vi "PilotPlant.vi"() -> ()   [LabVIEW 2015]
uses:
  <vilib>/addons/control/pid/NI_PID_pid.lvlib
  <vilib>/addons/control/pid/pid.llb/PID (DBL).vi
  state.ctl
  calcDoseorGetGraph.ctl
  data ave state.ctl
  Sensor buffer command.ctl
  file paths.ctl
  ini.ctl
  data channels.ctl
  coagbuffer.ctl
  model type.ctl
  Manual or Auto.ctl
  setpoints.ctl
  backwash.ctl
  coag.ctl
panel:
  in  "Tab Control":enum32{"Graphs", "Controls", "About"}(tab)
  out "coag":cluster{"time":timestamp[], "all coag in":dbl[]}(graph)
  out "Misc":cluster{timestamp[], dbl[]}[](graph)
  out "Turbidities":cluster{timestamp[], dbl[]}[](graph)
  out "Sludge valve":dbl(graph)
  out "Plant flow valve":dbl(graph)
  in  "data channel":T1
  out "recent data":dbl[](array[numeric])
  in  "setpoints":T2={"graph data interval (s)"=100.0, "sludge flow [L/s]"=0.0, "plant flow [L/s]"=0.05, "Plant Flow PID "={"proportional gain (Kc)"=0.05, "integral time (Ti, min)"=1.0, "derivative time (Td, min)"=0.01}, "Sludge PID "={"proportional gain (Kc)"=0.07, "integral time (Ti, min)"=1.0, "derivative time (Td, min)"=0.01}, "backwash"={"Filtered quality target [NTU]"=0.3, "min filtration time [s]"=600.0, "Ripen time [s]"=600.0}, "Coagulant"={"flocculator volume (L)"=0.0, "clarifier volume (L)"=0.0, "dose updates per HRT"=100, "target clarified turbidity (NTU)"=0.3, "Coagulant mode"=enum."manual", "Coag dose [mg/L]"=0.0, "pump mL/rev"=0.0, "clarifier flow [L/s]"=0.5, "min Coag dose [mg/L]"=0.0, "max Coag dose [mg/L]"=0.0, "Steps"=3, "HRT response delay"=1, "Ku*"=1.0}} {"Coagulant"."HRT response delay" min=1 max=10 step=1; "Coagulant"."Steps" min=3 step=1; "Coagulant"."clarifier flow [L/s]" min=0.0001 max=1.0 step=0.0001; "Coagulant"."target clarified turbidity (NTU)" min=0.1 max=5.0 step=0.01; "Coagulant"."dose updates per HRT" min=1 max=100 step=1; "Sludge PID"."derivative time (Td, min)" format="%.3f"; "Sludge PID"."integral time (Ti, min)" format="%.3f"; "Sludge PID"."proportional gain (Kc)" format="%.3f"; "Plant Flow PID"."derivative time (Td, min)" format="%.3f"; "Plant Flow PID"."integral time (Ti, min)" format="%.3f"; "Plant Flow PID"."proportional gain (Kc)" format="%.3f"; "plant flow [L/s]" min=0.05 max=1.0 step=0.05; "sludge flow [L/s]" min=0.0 max=0.05 step=0.001; "graph data interval (s)" min=1 max=1000 step=1}
  in  "Sludge valve [V]":dbl(slide)=1.5 scale=0.0..5.0
  in  "Sludge control":bool
  out "coag pump In Range?":bool
  out "coag model":T5
  in  "backwash [ON/OFF]":bool
  out "Last backwash":timestamp
  in  "Backwash control":T6
  out "error out":errorcluster
  out "total HRT":dbl
  out "coag dose [mg/L]":dbl
  out "rpm":dbl
  in  "channel":T1=enum."raw [NTU]"
  out "stopping":bool
  out "data labels":string[](array[string])
  in  "Shut Down":bool
  # "min"
  # "max"
  # "The coaglog saves the coagulant and turbidity values for that particular time. There is no offset to correct for HRT."
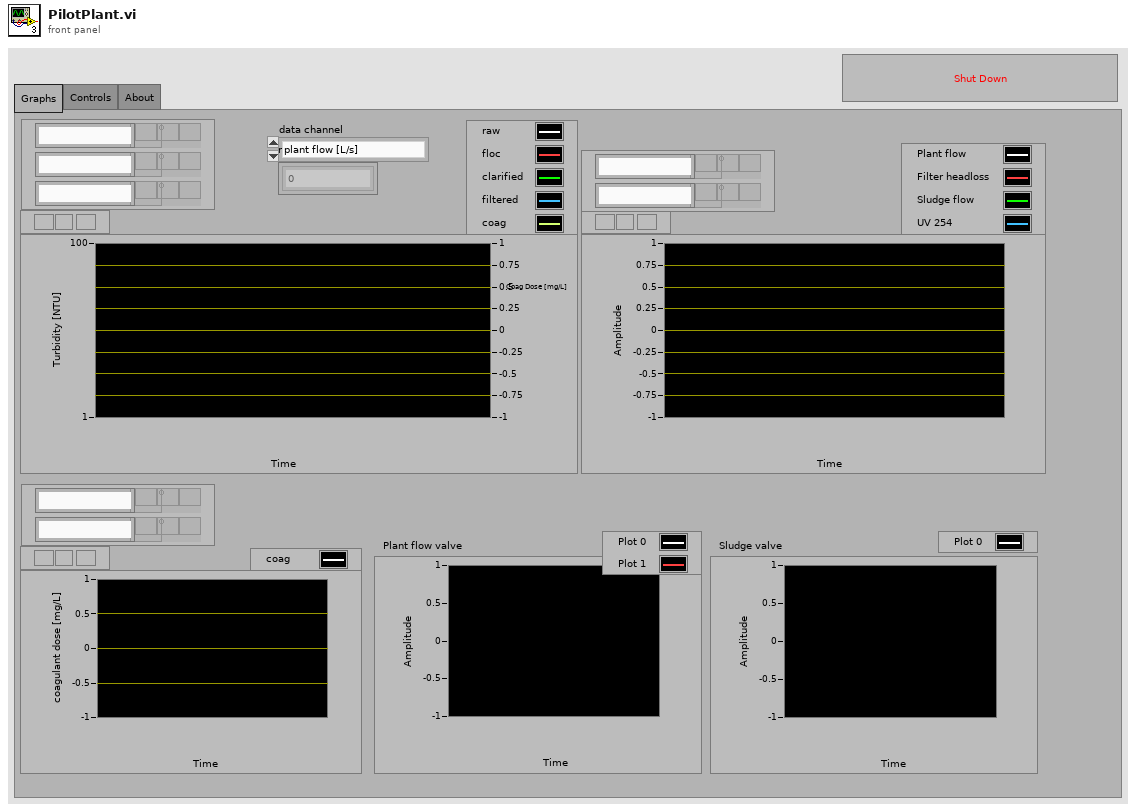
[diagram p1: front panel]
types:
  T1 = typedef "data channels.ctl" = enum16{"plant flow [L/s]", "Head Loss [m]", "sludge flow [L/s]", "UV 254", "raw [NTU]", "floc sed [NTU]", "clarified [NTU]", "filtered [NTU]"}
  T2 = typedef "setpoints.ctl" = cluster{"graph data interval (s)":sgl, "sludge flow [L/s]":dbl, "plant flow [L/s]":dbl, "Plant Flow PID ":cluster{"proportional gain (Kc)":dbl, "integral time (Ti, min)":dbl, "derivative time (Td, min)":dbl}, "Sludge PID ":cluster{"proportional gain (Kc)":dbl, "integral time (Ti, min)":dbl, "derivative time (Td, min)":dbl}, "backwash":T3, "Coagulant":T4}
  T3 = typedef "backwash.ctl" = cluster{"Filtered quality target [NTU]":dbl, "min filtration time [s]":dbl, "Ripen time [s]":dbl}
  T4 = typedef "coag.ctl" = cluster{"flocculator volume (L)":dbl, "clarifier volume (L)":dbl, "dose updates per HRT":u16, "target clarified turbidity (NTU)":dbl, "Coagulant mode":T5, "Coag dose [mg/L]":dbl, "pump mL/rev":dbl, "clarifier flow [L/s]":dbl, "min Coag dose [mg/L]":dbl, "max Coag dose [mg/L]":dbl, "Steps":u16, "HRT response delay":u32, "Ku*":dbl}
  T5 = typedef "model type.ctl" = enum16{"manual", "ramp", "simple corrector", "linear regression"}
  T6 = typedef "Manual or Auto.ctl" = enum16{"Manual", "Automatic"}
  T7 = typedef "file paths.ctl" = enum16{"read paths", "close"}
  T8 = typedef "ini.ctl" = enum16{"write", "read"}
  T9 = typedef "data ave state.ctl" = enum16{"Initialize", "Process data"}
  T10 = typedef "state.ctl" = enum16{"Initialize", "Process data", "Close"}
  T11 = typedef "Sensor buffer command.ctl" = enum16{"set buffer size", "write", "refill buffer", "read recent", "read all", "clear"}
  T12 = typedef "calcDoseorGetGraph.ctl" = enum16{"calculate dose", "read graph"}
  T13 = typedef "coagbuffer.ctl" = enum16{"set buffer size", "write", "refill buffer", "read recent", "read all", "clear", "overwrite"}
  T14 = typedef "data cluster.ctl" = cluster{"floc sed turbidity (NTU)":dbl, "Raw turbidity (NTU)":dbl, "flow rate (L/s)":dbl, "time":timestamp}
  T15 = cluster{"proportional gain (Kc)":dbl, "integral time (Ti, min)":dbl, "derivative time (Td, min)":dbl}
  T16 = cluster{"time":timestamp[], "all coag in":dbl[]}[]
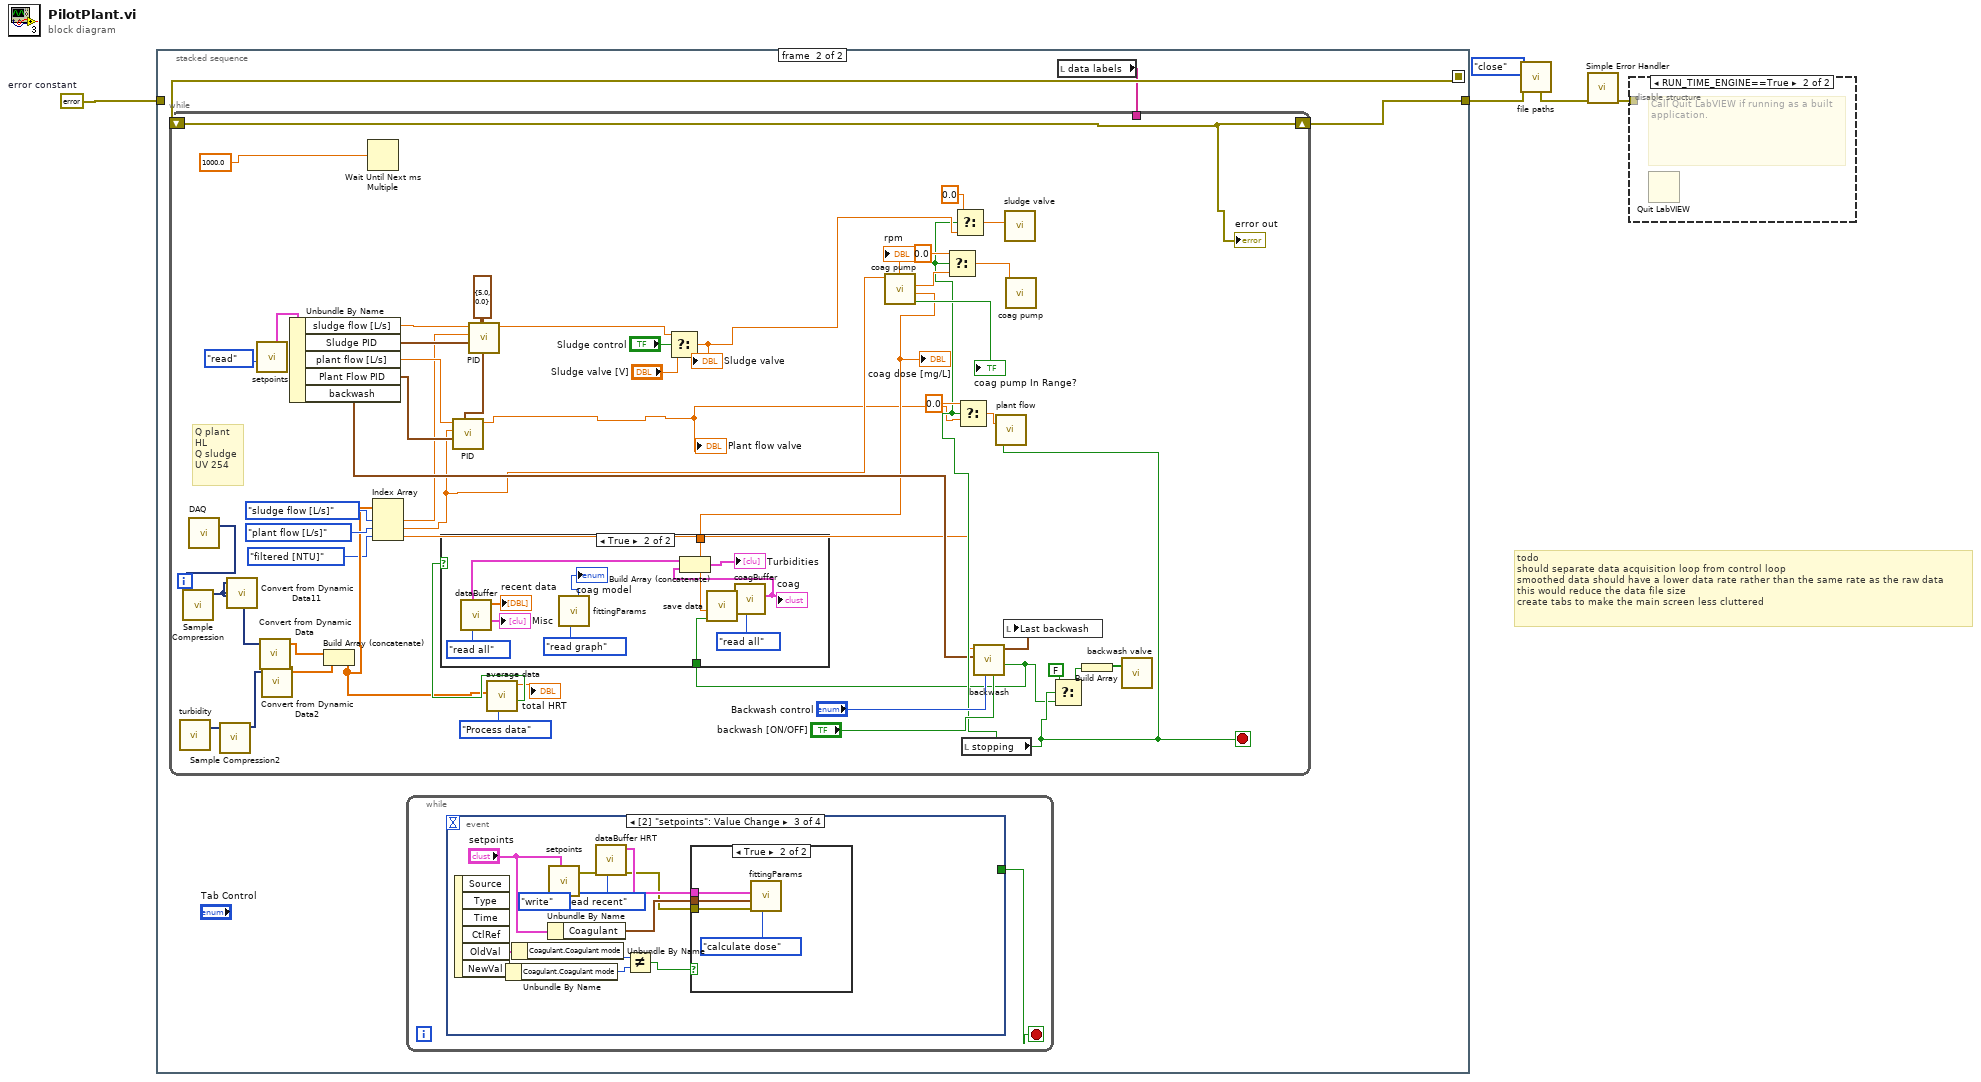
[diagram p0: block diagram]
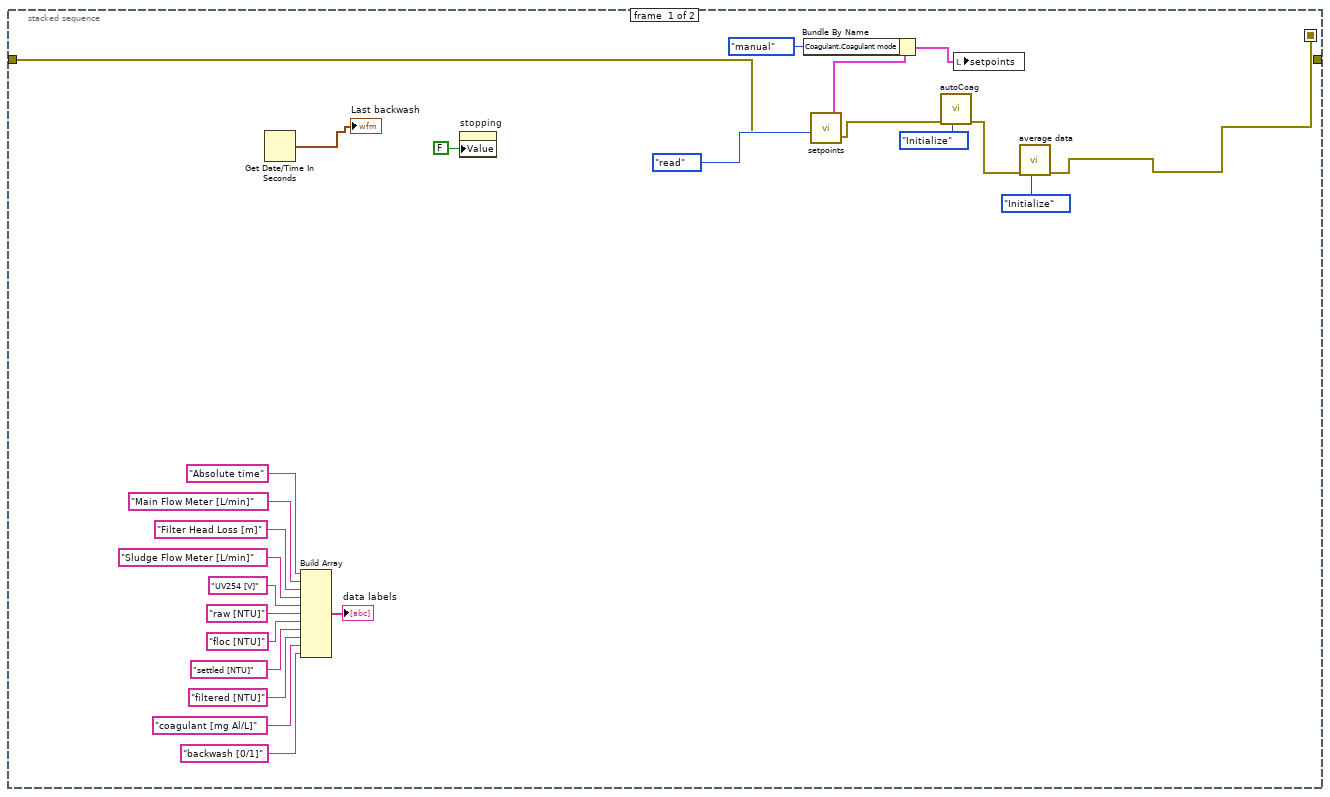
[diagram p2: hidden frame]
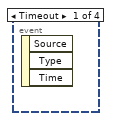
[diagram p3: hidden frame]
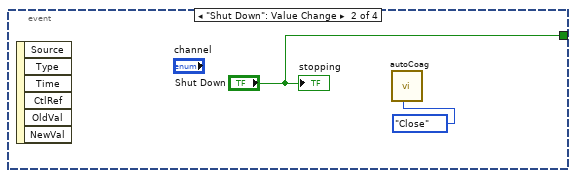
[diagram p4: hidden frame]
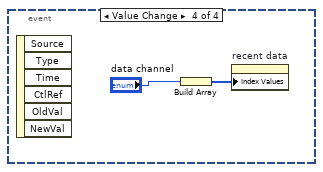
[diagram p6: hidden frame]
diagram:
  w5 = errorcluster {"status"=FALSE, "code"=0, "source"=""}  # error constant
  # "todo\nshould separate data acquisition loop from control loop\nsmoothed data should have a lower data rate rather than the same rate as the raw data\nthis would reduce the data file size\ncreate tabs to make the main screen less cluttered"
  n1 = stacked-sequence {
    seq-local: [w9 _] -> [_ w32]
    tunnel: w5 -> [w12 _]
    tunnel: [_ w30] -> w2
    frame #0 {
      n2 = Get Date/Time In Seconds() -> (seconds since 1Jan1904=→"Last backwash":timestamp)
      n3 = Build Array("Absolute time", "Main Flow Meter [L/min]", "Filter Head Loss [m]", "Sludge Flow Meter [L/min]", "UV254 [V]" ("element"), "raw [NTU]", "floc [NTU]", "settled [NTU]", "filtered [NTU]" ("element"), "coagulant [mg Al/L]" ("element"), "backwash [0/1]" ("element")) -> (→"data labels":string[])
      n4 = property on="stopping" class="Bool (strict)"("Value"=FALSE ("stopping")) -> ()  [unwired: 2 in, 2 out]
      n5 = call "setpoints.vi"("error in (no error)"=w12, "ini"=ini."read") -> ("error out"=w11:errorcluster, "Setpoints out"=w8:T2)  [unwired: 8 in]
      n6 = Bundle By Name(cluster=w8, "Coagulant.Coagulant mode"=model_type."manual") -> (w7:T2)
      n7 = call "autoCoag.vi"("state"=state."Initialize" ("Enum"), "error in (no error)"=w11) -> ("error out"=w14:errorcluster)  [unwired: 7 in, 2 out]
      n8 = local write "setpoints"(w7) -> ()
      n9 = call "average data.vi"("state"=data_ave_state."Initialize", "error in (no error)"=w14) -> ("error out"=w9:errorcluster)  [unwired: 5 in, 4 out]
    }
    frame #1 {
      n10 = while {
        stop <- w33 stop-if-true
        n11 = event shown="[2] \"setpoints\": Value Change" {
          selector: _ -> [_ _ _ _]
          dyn-events: _ -> [_ _ _ _]
          timeout: _ -> [_ _ _ _]
          tunnel: [_ "Shut Down" _ _] -> w33
          event Timeout {
            n12 = event-data() -> ()  [unwired: 1 in, 3 out]
          }
          event "Shut Down": Value Change {
            n13 = event-data() -> ()  [unwired: 1 in, 6 out]
            n14 = call "autoCoag.vi"("state"=state."Close" ("Enum")) -> ()  [unwired: 8 in, 3 out]
            "stopping" <- "Shut Down"
          }
          event Value Change {
            n15 = event-data() -> ("OldVal"=w39:T2, "NewVal"=w40:T2)  [unwired: 1 in, 4 out]
            n16 = Unbundle By Name(w40) -> ("Coagulant.Coagulant mode"=w37:T5)
            n17 = Unbundle By Name(w39) -> ("Coagulant.Coagulant mode"=w38:T5)
            n18 = Unbundle By Name("setpoints") -> ("Coagulant"=w45:T4)
            n19 = call "setpoints.vi"("setpoints"="setpoints", "ini"=ini."write") -> ("error out"=w42:errorcluster)  [unwired: 8 in, 1 out]
            n20 = call "dataBuffer HRT.vi"("command"=Sensor_buffer_command."read recent", "error in (no error)"=w42) -> ("error out"=w41:errorcluster, "recent data"=w44:T14)  [unwired: 6 in, 2 out]
            n21 = Not Equal?(x=w38, y=w37) -> (x != y?=w36:bool)
            n22 = case shown="True" w36 {
              tunnel: w45 -> [_ w51]
              tunnel: w44 -> [_ w49]
              tunnel: w41 -> [_ w48]
              frame False {
              }
              frame True {
                n23 = call "fittingParams.vi"("read/write"=calcDoseorGetGraph."calculate dose", "error in (no error)"=w48, "Coagulant"=w51, "averaged data"=w49) -> ()  [unwired: 5 in, 3 out]
              }
            }
          }
          event Value Change {
            n24 = event-data() -> ()  [unwired: 1 in, 6 out]
            n25 = Build Array("data channel") -> (w52:T1[])
            n26 = property on="recent data" class="Arr (strict)"("Index Values"=w52) -> ()  [unwired: 2 in, 2 out]
          }
        }
      }
      n27 = local read "data labels"() -> (w31:string[])
      n28 = while {
        shift-right: [w67] -> w30
        shift-left: w32 -> [w67]
        tunnel: w31 -> [_]
        stop <- w84 stop-if-true
        w97 = cluster{"output high":dbl, "output low":dbl} {"output high"=5.0, "output low"=0.0} ("output range")
        # "Q plant\nHL\nQ sludge\nUV 254"
        n29 = call "turbidity"() -> ("data"=w70:dynamicdata)  [unwired: 17 in, 2 out]
        n30 = call "DAQ"() -> ("data"=w71:dynamicdata)  [unwired: 17 in, 2 out]
        n31 = call "Sample Compression"("Signals"=w71) -> ("Mean"=w66:dynamicdata)  [unwired: 8 in, 2 out]
        n32 = call "Sample Compression2"("Signals"=w70) -> ("Mean"=w61:dynamicdata)  [unwired: 8 in, 2 out]
        n33 = call "Convert from Dynamic Data11"("Dynamic Data Type"=w66) -> ()  [unwired: 3 in, 1 out]
        n34 = call "setpoints.vi"("ini"=ini."read") -> ("Setpoints out"=w68:T2)  [unwired: 9 in, 1 out]
        n35 = call "Convert from Dynamic Data"("Dynamic Data Type"=w66) -> ("Array"=w82:dbl[])  [unwired: 3 in]
        n36 = call "Convert from Dynamic Data2"("Dynamic Data Type"=w61) -> ("Array"=w81:dbl[])  [unwired: 3 in]
        n37 = Unbundle By Name(w68) -> ("sludge flow [L/s]"=w77:dbl, "Sludge PID"=w76:T15, "plant flow [L/s]"=w75:dbl, "Plant Flow PID"=w74:T15, "backwash"=w73:T3)
        n38 = Build Array (concatenate)(w82, w81) -> (w60:dbl[])
        n39 = Wait Until Next ms Multiple(millisecond multiple=1000.0 ("y")) -> ()  [unwired: 1 out]
        n40 = Index Array(array=w60, index #1=data_channels."sludge flow [L/s]" ("channel"), index #2=data_channels."plant flow [L/s]" ("channel"), index #3=data_channels."filtered [NTU]" ("channel")) -> (element #1=w63:dbl, element #2=w62:dbl, element #3=w58:dbl)
        n41 = call-poly <vilib>:"PID.vi"("output range"=w97, "PID gains"=w74, "process variable"=w62, "setpoint"=w75) -> ("output"=w55:dbl)  [unwired: 6 in, 1 out]
        "Plant flow valve" <- w55
        n42 = call-poly <vilib>:"PID.vi"("output range"=w97, "PID gains"=w76, "process variable"=w63, "setpoint"=w77) -> ("output"=w98:dbl)  [unwired: 6 in, 1 out]
        n43 = call "average data.vi"("state"=data_ave_state."Process data", "data input"=w60) -> ("new interval"=w78:bool, "total HRT"=→"total HRT":dbl)  [unwired: 5 in, 3 out]
        n44 = Select(t=w98, s="Sludge control", f="Sludge valve [V]") -> (s? t:f=w88:dbl)
        "Sludge valve" <- w88
        n45 = call "coag pump.vi"("plant flow [L/s]"=w62) -> ("In Range?"=→"coag pump In Range?":bool, "coag dose [mg/L]"=w57:dbl, "pump [V]"=w93:dbl, "rpm"=→"rpm":dbl)  [unwired: 6 in, 1 out]
        "coag dose [mg/L]" <- w57
        n46 = local read "stopping"() -> (w84:bool)
        n47 = Select(t=0.0, s=w84, f=w93) -> (s? t:f=w92:dbl)
        n48 = Select(t=0.0, s=w84, f=w88) -> (s? t:f=w87:dbl)
        n49 = Select(t=0.0, s=w84, f=w55) -> (s? t:f=w91:dbl)
        n50 = call "backwash.vi"("Manual override"="backwash [ON/OFF]", "Backwash control"="Backwash control", "backwash"=w73, "Filtered Turbidity"=w58) -> ("backwashing?"=w56:bool, "last backwash"=w99:timestamp)  [unwired: 5 in, 1 out]
        n51 = case shown="True" w78 {
          tunnel: w57 -> [_ w109]
          tunnel: w56 -> [_ w108]
          frame False {
          }
          frame True {
            n52 = call "dataBuffer.vi"("command"=Sensor_buffer_command."read all") -> ("recent data"=→"recent data":dbl[], "misc graph"=→"Misc":cluster{timestamp[], dbl[]}[], "turbidity"=w112:cluster{timestamp[], dbl[]}[])  [unwired: 5 in, 3 out]
            n53 = call "fittingParams.vi"("read/write"=calcDoseorGetGraph."read graph") -> ("coag model"=→"coag model":T5)  [unwired: 8 in, 2 out]
            n54 = call "save data.vi"("backwashing?"=w108, "coagulant dose"=w109) -> ()  [unwired: 10 in]
            n55 = call "coagBuffer.vi"("command"=coagbuffer."read all") -> ("all data out"=w103:cluster{"time":timestamp[], "all coag in":dbl[]})  [unwired: 8 in, 2 out]
            "coag" <- w103
            n56 = Build Array (concatenate)(w112, w103) -> (→"Turbidities":T16)
          }
        }
        n57 = call "plant flow"("data"=w91, "stop (T)"=w84) -> ()  [unwired: 16 in, 2 out]
        n58 = local write "Last backwash"(w99) -> ()
        n59 = call "sludge valve"("data"=w87) -> ()  [unwired: 17 in, 2 out]
        n60 = call "coag pump"("data"=w92) -> ()  [unwired: 17 in, 2 out]
        n61 = Select(t=FALSE, s=w84, f=w56) -> (s? t:f=w85:bool)
        n62 = Build Array(w85) -> (w102:bool[])
        n63 = call "backwash valve"("data"=w102) -> ()  [unwired: 17 in, 2 out]
        "error out" <- w67
      }
    }
  }
  n64 = call "file paths.vi"("error in (no error)"=w2, "file path control"=file_paths."close") -> ("error out"=w1:errorcluster)  [unwired: 6 in, 3 out]
  n65 = call <vilib>:"Simple Error Handler.vi"("error in (no error)"=w1) -> ("error out"=w4:errorcluster)  [unwired: 4 in, 4 out]
  n66 = disable-structure shown="RUN_TIME_ENGINE==True" {
    disable-tunnel: w4 -> [_ _]
    frame condition #0 (active) {
    }
    frame condition #1 {
      # "Call Quit LabVIEW if running as a built application."
      n67 = Quit LabVIEW() -> ()  [unwired: 1 in]
    }
  }
